vi "Cleaned_Up_Final_Code_Balance.vi"() -> ()   [LabVIEW 2012]
uses:
  <vilib>/NXT/Subs/MotorOutput.ctl
  <vilib>/NXT/Block Support/NXT_TimerIndex.ctl
  <vilib>/NXT/Dual Mode Library/Display/drawText_Center.vi
  <vilib>/NXT/Dual Mode Library/Display/drawText.vi
panel:
  out "gyroSum":i16
  out "loop count":i32
  out "Gyro":i16
  out "power":dbl(graph)
  out "motorSpeed":dbl
  out "motorPos":i32
  out "motorDelta":i32(graph)
  out "motorSum":i32(graph)
  out "gyroAngle":dbl
  out "gyroSpeed":dbl
  out "gOffset":dbl
  out "tInterval":dbl
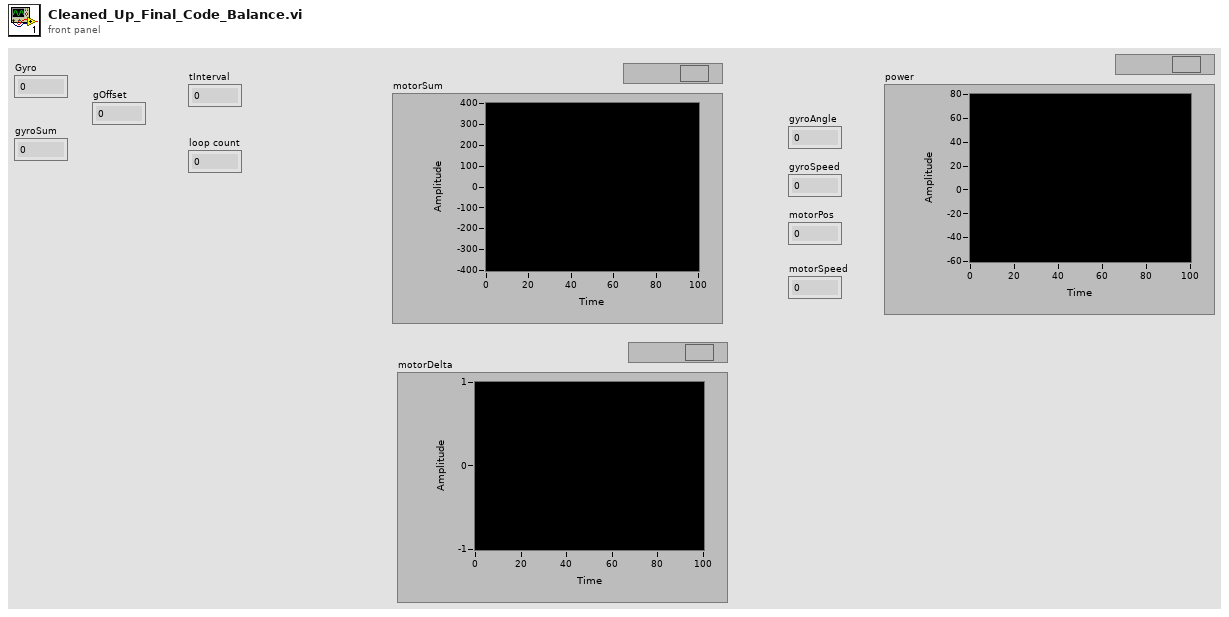
[diagram p1: front panel]
types:
  T1 = typedef "MotorOutput.ctl" = u8
  T2 = typedef "LVHSConnector.ctl" = cluster{"Hardware":string, "Flattened String":string}
  T3 = typedef "NXT_TimerIndex.ctl" = u8
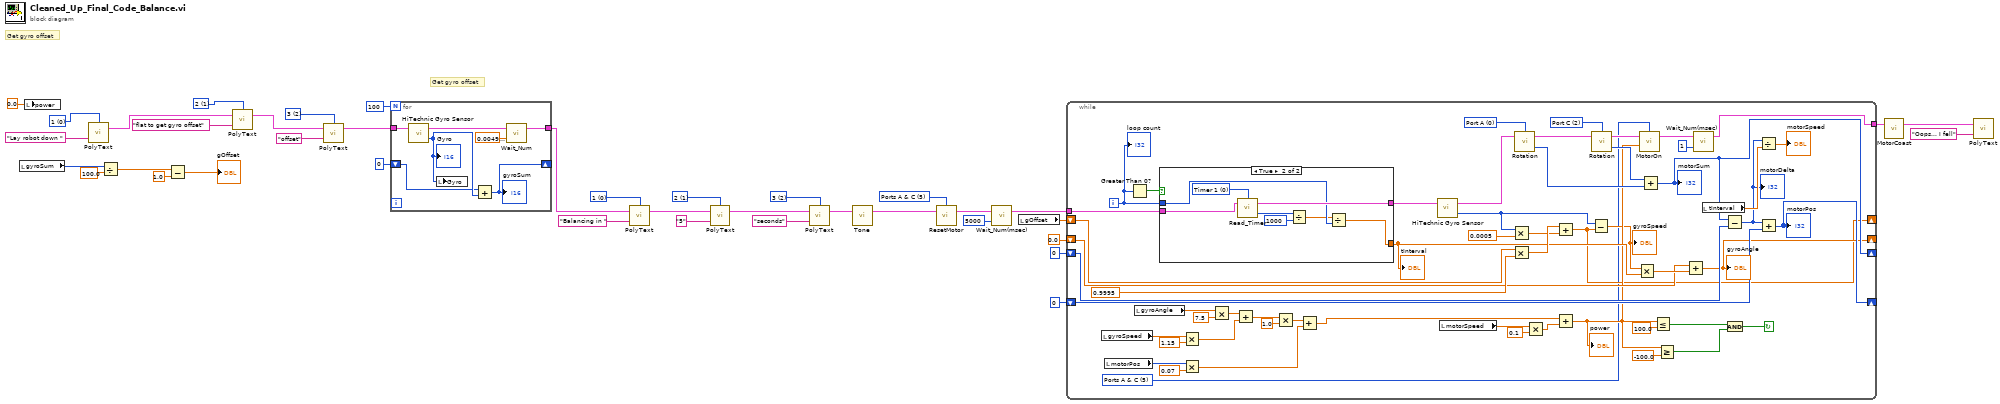
[diagram p0: block diagram]
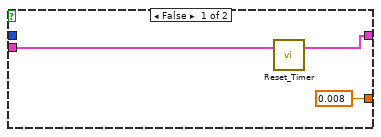
[diagram p2: hidden frame]
diagram:
  w7 = i16 0 items=["1", "2", "3", "4", "5", "6", "7", "8"] ("Line")
  w8 = i16 1 items=["1", "2", "3", "4", "5", "6", "7", "8"] ("Line")
  w9 = i16 2 items=["1", "2", "3", "4", "5", "6", "7", "8"] ("Line")
  w16 = i16 0 items=["1", "2", "3", "4", "5", "6", "7", "8"] ("Line")
  w17 = i16 1 items=["1", "2", "3", "4", "5", "6", "7", "8"] ("Line")
  w18 = i16 2 items=["1", "2", "3", "4", "5", "6", "7", "8"] ("Line")
  w37 = T1 5 items=["Port A"=0, "Port B"=1, "Port C"=2, "Ports A & B"=4, "Ports A & C"=5, "Ports B & C"=6, "All Ports"=3] ("Port (All Ports)")
  # "Get gyro offset"
  # "Get gyro offset"
  n1 = local read "gyroSum"() -> (w25:i16)
  n2 = local write "power"(0.0 ("power")) -> ()
  n3 = call-poly <vilib>:"PolyText.vi"("Text"="Lay robot down ", "Line"=w16) -> ("NXT"=w20:T2)  [unwired: 2 in]
  n4 = Divide(x=w25, y=100.0) -> (x/y=w31:dbl)
  n5 = Subtract(x=w31, y=1.0) -> (x-y=→"gOffset":dbl)
  n6 = call-poly <vilib>:"PolyText.vi"("Text"="flat to get gyro offset", "NXT"=w20, "Line"=w17) -> ("NXT"=w19:T2)  [unwired: 1 in]
  n7 = call-poly <vilib>:"PolyText.vi"("Text"="offset", "NXT"=w19, "Line"=w18) -> ("NXT"=w14:T2)  [unwired: 1 in]
  n8 = for {
    N: 100 -> [_]
    tunnel: [w44] -> w5
    shift-right: [w43] -> _
    shift-left: i16 0 -> [w42]
    tunnel: w14 -> [w41]
    n9 = call <vilib>:"HiTechnic Gyro Sensor.vi"("NXT"=w41) -> ("Gyro Value"=w46:i16, "NXT"=w40:T2)  [unwired: 2 in]
    "Gyro" <- w46
    n10 = local write "Gyro"(w46) -> ()
    n11 = Add(x=w42, y=w46) -> (x+y=w43:i16)
    "gyroSum" <- w43
    n12 = call <vilib>:"Wait_Num.vi"("Time (1 sec)"=sgl 0.005, "NXT"=w40) -> ("NXT"=w44:T2)  [unwired: 2 in]
  }
  n13 = call-poly <vilib>:"PolyText.vi"("Text"="Balancing in ", "NXT"=w5, "Line"=w7) -> ("NXT"=w11:T2)  [unwired: 1 in]
  n14 = call-poly <vilib>:"PolyText.vi"("Text"="5", "NXT"=w11, "Line"=w8) -> ("NXT"=w10:T2)  [unwired: 1 in]
  n15 = call-poly <vilib>:"PolyText.vi"("Text"="seconds", "NXT"=w10, "Line"=w9) -> ("NXT"=w4:T2)  [unwired: 1 in]
  n16 = call <vilib>:"Tone.vi"("NXT"=w4) -> ("NXT"=w34:T2)  [unwired: 3 in]
  n17 = call <vilib>:"ResetMotor.vi"("NXT"=w34, "Port (All Ports)"=w37) -> ("NXT"=w36:T2)  [unwired: 2 in]
  n18 = call <vilib>:"Wait_Num(msec).vi"("Time (100 msec)"=u32 5000, "NXT"=w36) -> ("NXT"=w35:T2)  [unwired: 2 in]
  n19 = local read "gOffset"() -> (w2:dbl)
  n20 = while {
    tunnel: w35 -> [w70]
    shift-right: [w69] -> _
    shift-left: 0 -> [w68]
    shift-right: [w65] -> _
    shift-left: 0 -> [w67]
    shift-right: [w55] -> _
    shift-left: 0.0 -> [w54]
    tunnel: [w50] -> w24
    shift-right: [w51] -> _
    shift-left: w2 -> [w64]
    i -> [w61]
    stop <- w47 continue-if-true
    w49 = T1 5 items=["Port A"=0, "Port B"=1, "Port C"=2, "Ports A & B"=4, "Ports A & C"=5, "Ports B & C"=6, "All Ports"=3] ("Output Port (All Ports)")
    w92 = u8 2 items=["Port A", "Port B", "Port C"] ("Port (Port A)")
    w93 = u8 0 items=["Port A", "Port B", "Port C"] ("Port (Port A)")
    n21 = local read "gyroSpeed"() -> (w58:dbl)
    n22 = local read "motorPos"() -> (w57:i32)
    n23 = Greater Than 0?(x=w61) -> (x > 0?=w62:bool)
    n24 = local read "gyroAngle"() -> (w63:dbl)
    n25 = case shown="True" w62 {
      tunnel: [w105 w113] -> w102
      tunnel: w70 -> [w104 w112]
      tunnel: [0.008 ("tInterval") w111] -> w60
      tunnel: w61 -> [_ w109]
      frame False {
        n26 = call <vilib>:"Reset_Timer.vi"("NXT"=w104) -> ("NXT"=w105:T2)  [unwired: 3 in]
      }
      frame True {
        w110 = T3 0 items=["Timer 1", "Timer 2", "Timer 3"] ("Timer (Timer 1)")
        n27 = call <vilib>:"Read_Timer.vi"("NXT"=w112, "Timer (Timer 1)"=w110) -> ("Value (msec)"=w108:u32, "NXT"=w113:T2)  [unwired: 1 in]
        n28 = Divide(x=w108, y=u32 1000) -> (x/y=w106:dbl)
        n29 = Divide(x=w106, y=w109) -> (x/y=w111:dbl)
      }
    }
    "tInterval" <- w60
    n30 = Multiply(x=w58, y=1.15) -> (x*y=w86:dbl)
    n31 = Multiply(x=w57, y=0.07) -> (x*y=w80:dbl)
    n32 = Multiply(x=w63, y=7.5) -> (x*y=w87:dbl)
    n33 = Add(x=w87, y=w86) -> (x+y=w85:dbl)
    n34 = Multiply(x=w85, y=1.0) -> (x*y=w81:dbl)
    n35 = Add(x=w81, y=w80) -> (x+y=w79:dbl)
    n36 = call <vilib>:"HiTechnic Gyro Sensor.vi"("NXT"=w102) -> ("Gyro Value"=w97:i16, "NXT"=w95:T2)  [unwired: 2 in]
    n37 = local read "motorSpeed"() -> (w56:dbl)
    n38 = Multiply(x=w97, y=0.0005) -> (x*y=w98:dbl)
    n39 = Multiply(x=w64, y=0.9995) -> (x*y=w99:dbl)
    n40 = call <vilib>:"Rotation.vi"("NXT"=w95, "Port (Port A)"=w93) -> ("Angle of Rotation"=w90:i32, "NXT"=w94:T2)  [unwired: 1 in]
    n41 = Multiply(x=w56, y=0.1) -> (x*y=w78:dbl)
    n42 = Add(x=w99, y=w98) -> (x+y=w51:dbl)
    n43 = Add(x=w79, y=w78) -> (x+y=w53:dbl)
    "power" <- w53
    n44 = Subtract(x=w97, y=w51) -> (x-y=w52:dbl)
    "gyroSpeed" <- w52
    n45 = call <vilib>:"Rotation.vi"("NXT"=w94, "Port (Port A)"=w92) -> ("Angle of Rotation"=w91:i32, "NXT"=w77:T2)  [unwired: 1 in]
    n46 = Multiply(x=w52, y=w60) -> (x*y=w96:dbl)
    n47 = call <vilib>:"MotorOn.vi"("Power (75)"=w53, "NXT"=w77, "Output Port (All Ports)"=w49) -> ("NXT"=w76:T2)  [unwired: 1 in]
    n48 = Add(x=w91, y=w90) -> (x+y=w69:i32)
    "motorSum" <- w69
    n49 = Less Or Equal?(x=w53, y=100.0) -> (x <= y?=w72:bool)
    n50 = Greater Or Equal?(x=w53, y=-100.0) -> (x >= y?=w71:bool)
    n51 = Add(x=w54, y=w96) -> (x+y=w55:dbl)
    "gyroAngle" <- w55
    n52 = call <vilib>:"Wait_Num(msec).vi"("Time (100 msec)"=u32 1, "NXT"=w76) -> ("NXT"=w50:T2)  [unwired: 2 in]
    n53 = local read "tInterval"() -> (w59:dbl)
    n54 = Subtract(x=w69, y=w68) -> (x-y=w48:i32)
    "motorDelta" <- w48
    n55 = And(x=w72, y=w71) -> (x .and. y?=w47:bool)
    n56 = Divide(x=w48, y=w59) -> (x/y=→"motorSpeed":dbl)
    n57 = Add(x=w48, y=w67) -> (x+y=w65:i32)
    "motorPos" <- w65
    "loop count" <- w61
  }
  n58 = call <vilib>:"MotorCoast.vi"("NXT"=w24) -> ("NXT"=w39:T2)  [unwired: 3 in]
  n59 = call-poly <vilib>:"PolyText.vi"("Text"="Oops... I fell", "NXT"=w39) -> ()  [unwired: 2 in, 1 out]
